vi "读取通信状态.vi"(8 "error in (no error)":errorcluster, 11 "串口通信类 in":refnum<class "串口通信类.lvclass">) -> (0 "error out":errorcluster, 2 "通信状态":T1, 3 "串口通信类 out":refnum<class "串口通信类.lvclass">)   [LabVIEW 2015, in "串口通信类.lvclass"]
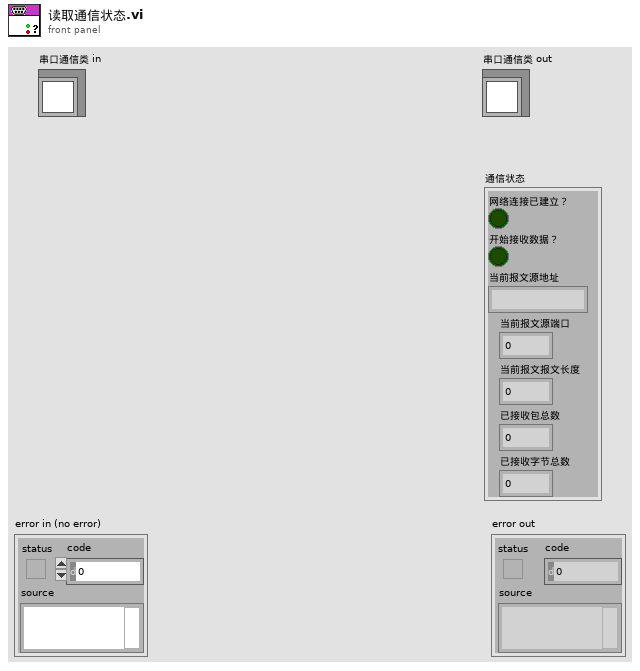
[diagram p1: front panel]
types:
  T1 = cluster{"网络连接已建立？":bool, "开始接收数据？":bool, "当前报文源地址":string, "当前报文源端口":u16, "当前报文报文长度":i32, "已接收包总数":u64, "已接收字节总数":u64}
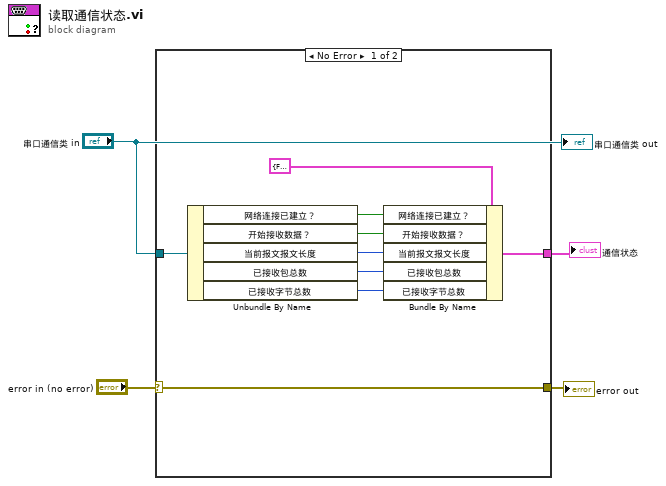
[diagram p0: block diagram]
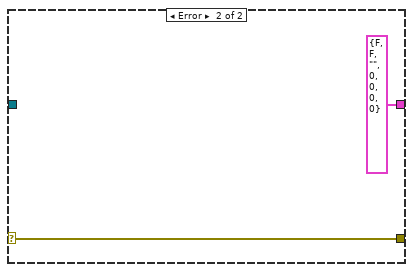
[diagram p2: hidden frame]
diagram:
  n1 = case shown="No Error" "error in (no error)" {
    selector: "error in (no error)" -> [w5 w15]
    tunnel: "串口通信类 in" -> [w13 _]
    tunnel: [w6 T1 {"网络连接已建立？"=FALSE, "开始接收数据？"=FALSE, "当前报文源地址"="", "当前报文源端口"=0, "当前报文报文长度"=0, "已接收包总数"=0, "已接收字节总数"=0} ("通信状态")] -> w3
    tunnel: [w5 w15] -> w1
    frame No Error {
      n2 = Unbundle By Name(w13) -> ("网络连接已建立？"=w11:bool, "开始接收数据？"=w10:bool, "当前报文报文长度"=w9:i32, "已接收包总数"=w8:u64, "已接收字节总数"=w7:u64)
      n3 = Bundle By Name(cluster=T1 {"网络连接已建立？"=FALSE, "开始接收数据？"=FALSE, "当前报文源地址"="", "当前报文源端口"=0, "当前报文报文长度"=0, "已接收包总数"=0, "已接收字节总数"=0} ("通信状态"), "网络连接已建立？"=w11, "开始接收数据？"=w10, "当前报文报文长度"=w9, "已接收包总数"=w8, "已接收字节总数"=w7) -> (w6:T1)
    }
    frame Error {
    }
  }
  "error out" <- w1
  "通信状态" <- w3
  "串口通信类 out" <- "串口通信类 in"
